vi "Curved Pulses.vi"() -> ()   [LabVIEW 2020]
uses:
  <vilib>/Analysis/1siggen.llb/Ramp Pattern by Samples.vi
  <vilib>/Analysis/3filter.llb/IIR Filter (DBL).vi
  <vilib>/Analysis/3filter.llb/FIR Filter (DBL).vi
  <vilib>/Analysis/NI_AALBase.lvlib
panel:
  out "sum 2":dbl
  out "sum":dbl
  out "Waveform Graph":waveform(dbl)[](graph)
  in  "Plateau Time (s)":dbl
  in  "Curve Parameter":dbl
  in  "Ramp Time (s)":dbl
  in  "Amplitude (mA)":dbl
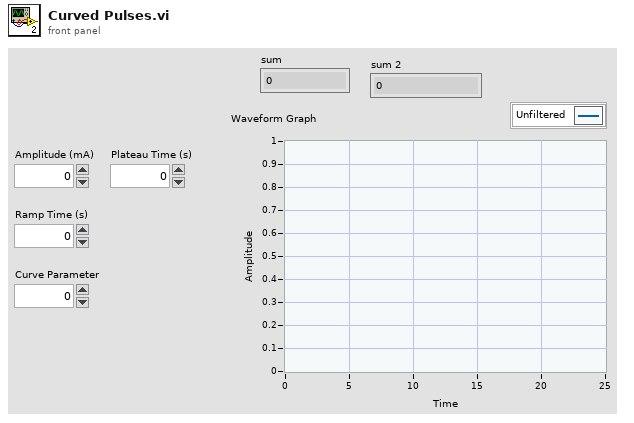
[diagram p1: front panel]
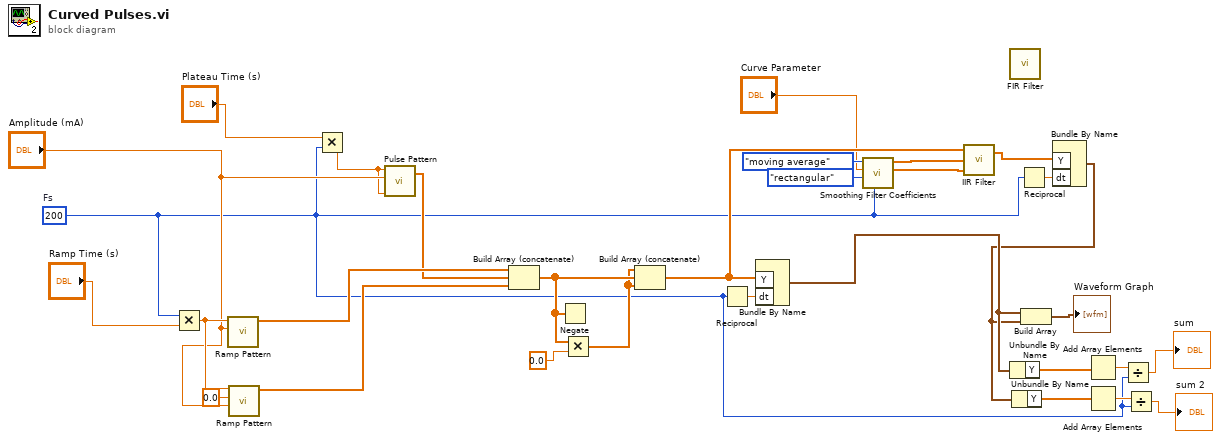
[diagram p0: block diagram]
diagram:
  w2 = 200  # Fs
  n1 = Multiply(x=w2, y="Ramp Time (s)") -> (x*y=w29:dbl)
  n2 = call-poly <vilib>:"Ramp Pattern.vi"("end"="Amplitude (mA)", "samples"=w29) -> ("Ramp Pattern"=w25:dbl[])  [unwired: 8 in, 1 out]
  n3 = call-poly <vilib>:"Ramp Pattern.vi"("start"="Amplitude (mA)", "end"=0.0, "samples"=w29) -> ("Ramp Pattern"=w24:dbl[])  [unwired: 7 in, 1 out]
  n4 = Multiply(x="Plateau Time (s)", y=w2) -> (x*y=w21:dbl)
  n5 = call <vilib>:"Pulse Pattern.vi"("width"=w21, "amplitude"="Amplitude (mA)", "samples"=w21) -> ("Pulse Pattern"=w23:dbl[])  [unwired: 1 in, 1 out]
  n6 = Build Array (concatenate)(w25, w23, w24) -> (w19:dbl[])
  n7 = Negate(x=w19) -> ()  [unwired: 1 out]
  n8 = Multiply(x=w19, y=0.0) -> (x*y=w15:dbl[])
  n9 = Build Array (concatenate)(w15, w19, w15) -> (w8:dbl[])
  n10 = Reciprocal(x=w2) -> (1/x=w26:dbl)
  n11 = Bundle By Name("Y"=w8, "dt"=w26) -> (w18:waveform(dbl))  [unwired: 1 in]
  n12 = call <vilib>:"Smoothing Filter Coefficients.vi"("fs"=w2, "shape"=enum16{"rectangular", "triangular"}."rectangular", "half-width"="Curve Parameter", "type"=enum16{"moving average", "exponential"}."moving average") -> ("forward coefficients"=w9:dbl[], "reverse coefficients"=w10:dbl[])  [unwired: 5 in, 1 out]
  n13 = call-poly <vilib>:"IIR Filter.vi"("Forward Coefficients"=w9, "Reverse Coefficients"=w10, "X"=w8) -> ("Filtered X"=w3:dbl[])  [unwired: 1 in, 1 out]
  n14 = call-poly <vilib>:"FIR Filter.vi"() -> ()  [unwired: 4 in, 2 out]
  n15 = Unbundle By Name(w18) -> ("Y"=w16:dbl[])
  n16 = Reciprocal(x=w2) -> (1/x=w4:dbl)
  n17 = Bundle By Name("Y"=w3, "dt"=w4) -> (w1:waveform(dbl))  [unwired: 1 in]
  n18 = Unbundle By Name(w1) -> ("Y"=w17:dbl[])
  n19 = Build Array(w18, w1) -> (→"Waveform Graph":waveform(dbl)[])
  n20 = Add Array Elements(numeric array=w16) -> (sum=w14:dbl)
  n21 = Add Array Elements(numeric array=w17) -> (sum=w13:dbl)
  n22 = Divide(x=w14, y=w2) -> (x/y=→"sum":dbl)
  n23 = Divide(x=w13, y=w2) -> (x/y=→"sum 2":dbl)
